vi "Test Get Failed Items Does Not Include Tests Not Executed.vi"(8 "error in (no error)":errorcluster, 11 "Result Model Result Recording Test in":refnum<class "Result Model Result Recording Test.lvclass">) -> (0 "error out":errorcluster, 3 "Result Model Result Recording Test out":refnum<class "Result Model Result Recording Test.lvclass">)   [LabVIEW 2020, in "Result Model Result Recording Test.lvclass"]
uses:
  Result Model Result Recording Test.lvclass
  C:/Program Files (x86)/National Instruments/LabVIEW 2020/vi.lib/Astemes/LUnit/Test Case.lvclass
  source/User Interface/Result Model/Tree Item Filter.ctl
  <vilib>/Astemes/LUnit/Test Case.lvclass/Test Case.ctl
  ae2c71b8-32bb-49d1-8500-0119bfec74ff.vi
  <vilib>/Astemes/LUnit/Append Pass Result.vi
  <vilib>/Astemes/LUnit/Append Fail Result.vi
  <vilib>/Astemes/LUnit/Describe Comparison.vi
  <vilib>/Astemes/LUnit/Compare Variants.vi
  <vilib>/Astemes/LUnit/Variant to string.vi
  <vilib>/Utility/Data Type/Get Type Information.vi
  <vilib>/Utility/LVClass/Get LV Class Name.vi
  Result Model Result Recording Test.lvclass/Result Model Result Recording Test.ctl
  source/User Interface/Result Model by Reference/Result Model by Reference.lvclass
  source/User Interface/Result Model/Result Model.lvclass
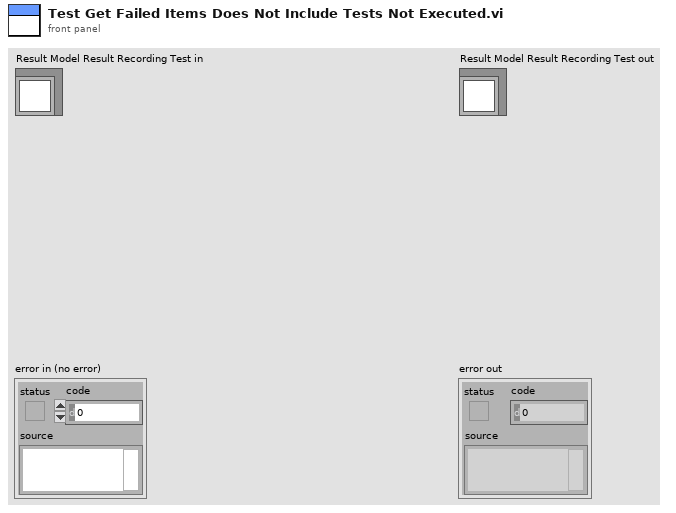
[diagram p1: front panel]
types:
  T1 = typedef "Result Model.lvclass/Tree Item Filter.ctl" = enum16{"All", "Only Fails", "Fails and Not Executed"}
  T2 = cluster{"Left Cell String":string, "Child Text":string[], "Child Tag":string, "Item Indent":i32, "Child Only?":bool, "Glyph Index":i32}[]
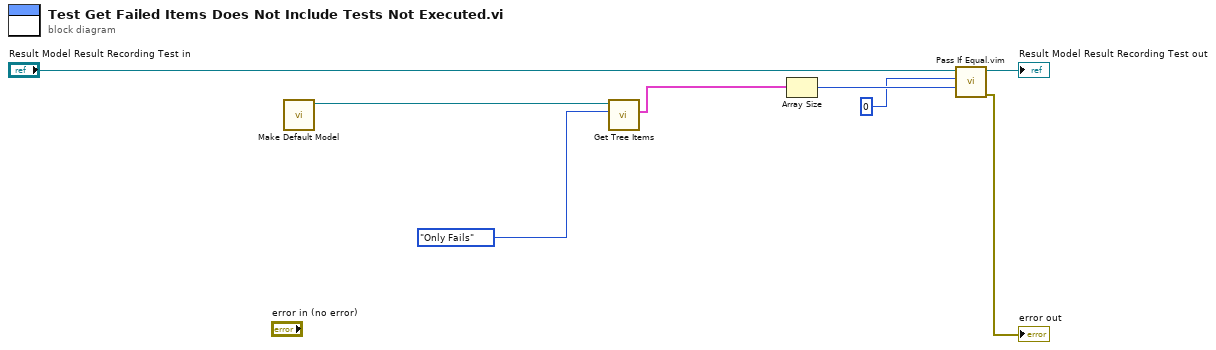
[diagram p0: block diagram]
diagram:
  n1 = call "Make Default Model.vi"() -> ("Result Model out"=w8:refnum<class "Result Model by Reference.lvclass">)  [unwired: 10 in, 1 out]
  n2 = call "Get Tree Items.vi"("Filter"=Tree_Item_Filter."Only Fails", "Result Model by Reference In"=w8) -> ("Tree Items"=w7:T2)  [unwired: 8 in, 1 out]
  n3 = Array Size(array=w7) -> (size(s)=w3:i32)
  n4 = call "Pass If Equal.vim"("Actual"=w3, "Expected"=0 ("size(s)"), "LUnit Test Case In"="Result Model Result Recording Test in") -> ("error out"=→"error out":errorcluster, "LUnit Test Case Out"=→"Result Model Result Recording Test out":refnum<class "Result Model Result Recording Test.lvclass">)  [unwired: 7 in]
